vi "Dashboard Main.vi"() -> ()   [LabVIEW 2013]
uses:
  Vision Processing/TargetType.ctl
  <vilib>/event_ctls.llb/eventvkey.ctl
  <vilib>/Rock Robotics/WPI/Dashboard/WPI_DashboardLogging Global.vi
  <vilib>/Utility/config.llb/Write Key (String).vi
  <vilib>/Utility/config.llb/Write Key (I32).vi
  <vilib>/Utility/config.llb/NI_LVConfig.lvlib
panel:
  out "Image Message":string="Timeout in Camera Communications"
  in  "Rec Mode":enum32{"Stop", "Record", "Playback"}(radio)
  in  "Dashboard Tab":T1(tab)
  in  "Idle Loader":bool
  out "Charged":bool=TRUE
  out "60 PSI":bool
  out "PSI":dbl format="%#_3g"
  out "One Driver":bool
  out "120 PSI":bool
  out "Trigger Locked":bool=TRUE
  out "Reverse Drive":bool
  out "Robot Velocity (ft/s)":dbl(slide) scale=-20.0..20.0
  out "Gyro Mode":bool
  out "GREEN":bool
  out "YELLOW":bool
  out "RED":bool=TRUE
  out "Distance (ft)":dbl
  in  "Camera Settings":T2={"Frame Rate"=30, "Compression"=30, "Size"=1} {"Frame Rate" scale=1.0..30.0; "Size" items=["640x480", "320x240", "160x120"]}
  out "MotorSliders R":cluster{"MotorSlide1":dbl, "MotorSlide2":dbl} {"MotorSlide2" scale=-1.0..1.0 scale format="%#_2e"; "MotorSlide1" scale=-1.0..1.0 scale format="%#_2e"}
  out "MotorChart R":cluster{"Numeric":dbl, "Numeric":dbl}(graph)
  out "MotorSliders L":T3 {"MotorSlide4 2" scale=0.0..14.0 scale format="%#_2e"; "MotorSlide2" scale=-1.0..1.0 scale format="%#_2e"; "MotorSlide1" scale=-1.0..1.0 scale format="%#_2e"}
  out "MotorChart L":T4(graph)
  out "JS1 Z":dbl(slide) scale=-1.0..1.0 scale format="%#_2e"
  out "Joystick 1":cluster{"X":dbl, "Y":dbl}[](graph)
  out "JS Buttons 1":T5
  out "JS2 Z":dbl(slide) scale=-1.0..1.0 scale format="%#_2e"
  out "Joystick 2":cluster{"X":dbl, "Y":dbl}[](graph)
  out "JS Buttons 2":T5
  out "Mode":T6(ring)=enum."Auto Disabled"
  out "Camera IP":string
  in  "DB Camera Config":bool
  out "fps":dbl format="%#.1g"
  out "Mbps":dbl format="%#.1g"
  out "Mbps 2":bool
  out "Angular Rate":dbl
  out "Gyro Angle":dbl
  in  "Automatic or Timed":bool
  out "HOT OR NOT":bool
  in  "Score Limit":dbl=60.0
  in  "Color Components":T7={"Hue"={69.0, 101.0}, "Sat"={160.89285714285714, 255.0}, "Val"={36.42857142857143, 230.7142857142857}} {"Val" scale=0.0..255.0; "Sat" scale=0.0..255.0; "Hue" scale=0.0..255.0 scale format="%#_3g"}
  out "Distances":T9(array[cluster])
  in  "Test Slider":dbl(slide) scale=0.0..100.0 scale format="%#_3g"
  in  "On/Off":bool caption="Solenoid"
  in  "Test Name":u16(ring) items=["Select the test to run...", "Example Test", "-------------------------------", "List of tests is built in robot code.", "Replace with your own automated tests."]
  in  "Test Tree":string(tree)
  in  "Motor":cluster{"Value":dbl, "Enable":bool} {"Value" scale=-1.0..1.0 scale format="%#_3g"}
  out "Progress":T10 {"Test Progress" scale=0.0..100.0}
  in  "Rev/Fwd":cluster{"Forward":bool, "Reverse":bool}
  in  "Test Ring":u16(ring) items=["Auto", "Fixed indoor", "Fixed outdoor 1", "Fixed outdoor 2", "Fixed fluorescent 1", "Fixed fluorescent 2", "Hold current"]
  in  "Listbox":i32(listbox)
  out "Tree":string(tree)
  out "Camera Image":T11(plugin-control)
  in  "Enable Vision":bool=TRUE
  # "Left"
  # "Front"
  # "Right"
  # "Battery"
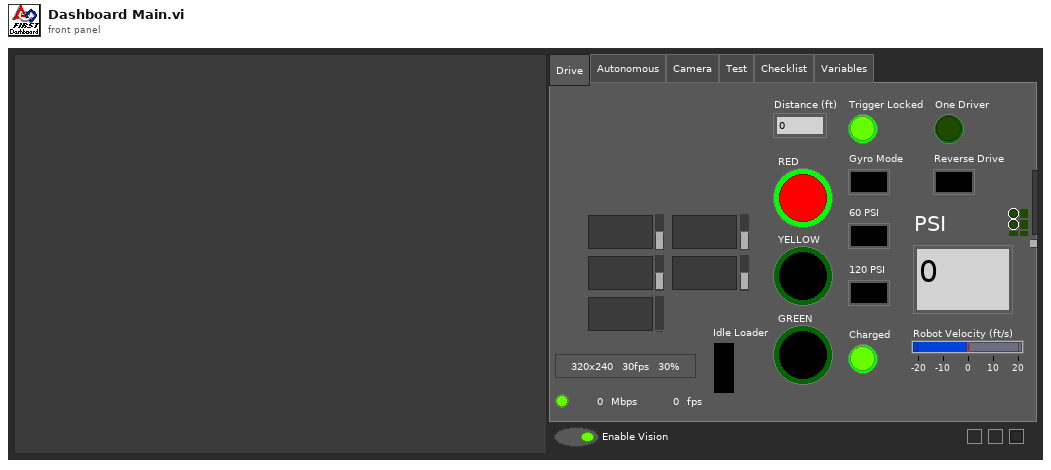
[diagram p1: front panel]
types:
  T1 = enum32{"Drive", "Autonomous", "Camera", "Test", "Checklist", "Variables"}
  T2 = cluster{"Frame Rate":i32, "Compression":i32, "Size":u16}
  T3 = cluster{"MotorSlide1":dbl, "MotorSlide2":dbl, "MotorSlide4 2":dbl}
  T4 = cluster{"Numeric":dbl, "Numeric":dbl, "Battery":sgl}
  T5 = cluster{bool, bool, bool, bool, bool, bool, bool, bool, bool, bool, bool, bool}
  T6 = enum8{"Tele-Op Disabled", "Tele-Op Enabled", "Auto Disabled", "Auto Enabled", "Test Disabled", "Test Enabled", ""}
  T7 = cluster{"Hue":cluster{dbl, dbl}, "Sat":cluster{dbl, dbl}, "Val":cluster{dbl, dbl}}
  T8 = typedef "TargetType.ctl" = enum16{"Not Hot", "Hot"}
  T9 = cluster{"Distance (ft)":dbl, "Target Center (-1 to 1)":cluster{"X":dbl, "Y":dbl}, "Left":bool, "State":T8}[]
  T10 = cluster{"Test Progress":u8, "Test Progress Text":string}
  T11 = typedef "IMAQ Image.ctl" = refnum<image>
  T12 = enum32{"Drive", "Operation", "Auto", "Test", "Checklist", "Variables"}
  T13 = typedef "Image Type" = u32
  T14 = cluster{"Digital Inputs":bool[], "Digital Outputs":bool[]}
  T15 = cluster{"Competition mode":bool, "Robot Link":bool, "Autonomous":bool, "Enabled":bool, "E-Stop":bool, "Simulated":bool, "TestMode":bool, "Docked Window":bool}
  T16 = cluster{"Boolean Array[0]":bool, "Boolean Array[1]":bool, "Boolean Array[2]":bool, "Boolean Array[3]":bool, "Boolean Array[4]":bool, "Boolean Array[5]":bool, "Boolean Array[6]":bool, "Boolean Array[7]":bool, "Boolean Array[8]":bool, "Boolean Array[9]":bool, "Boolean Array[10]":bool, "Boolean Array[11]":bool}
  T17 = cluster{cluster{dbl, dbl}, cluster{dbl, dbl}, cluster{dbl, dbl}}
  T18 = cluster{"Horizontal":bool, "Aspect Score":dbl, "Rect Score":dbl, cluster{"Left":dbl, "Top":dbl, "Right":dbl, "Bottom":dbl}, "Equiv H":dbl, "Equiv V":dbl}[]
  T19 = cluster{"Scores":cluster{"Total":dbl, "Left":dbl, "Right":dbl, "Ratio":dbl, "Vertical":dbl, "index":i32, "State":T8}, "Verticals":cluster{"Horizontal?":bool, "Aspect Score":dbl, "Rect Score":dbl, cluster{"Left":dbl, "Top":dbl, "Right":dbl, "Bottom":dbl}, "Equiv H":dbl, "Equiv V":dbl}, "Horizontals":cluster{"Horizontal?":bool, "Aspect Score":dbl, "Rect Score":dbl, cluster{"Left":dbl, "Top":dbl, "Right":dbl, "Bottom":dbl}, "Equiv H":dbl, "Equiv V":dbl}, "Validated":bool}[]
  T20 = cluster{"Scores":cluster{"Total":dbl, "Left":dbl, "Right":dbl, "Ratio":dbl, "Vertical":dbl, "index":i32, "State":T8}, "Verticals":cluster{"Horizontal?":bool, "Aspect Score":dbl, "Rect Score":dbl, cluster{"Left":dbl, "Top":dbl, "Right":dbl, "Bottom":dbl}, "Equiv H":dbl, "Equiv V":dbl}, "Horizontals":cluster{"Horizontal?":bool, "Aspect Score":dbl, "Rect Score":dbl, cluster{"Left":dbl, "Top":dbl, "Right":dbl, "Bottom":dbl}, "Equiv H":dbl, "Equiv V":dbl}, "Distance (ft)":dbl, "Target Center (-1 to 1)":cluster{"X":dbl, "Y":dbl}}[]
  T21 = cluster{"Distance (ft)":dbl, "Target Center (-1 to 1)":cluster{"X":dbl, "Y":dbl}, "Left":bool, "State":T8}
  T22 = typedef "NI_LVConfig.lvlib/Config Data RefNum.ctl" = refnum<k1>
  T23 = typedef "eventvkey.ctl" = enum16{"ASCII", "Enter", "Return", "Shift", "Ctrl", "Alt", "Cmd", "Opt", "Caps", "NumLock", "Clear", "Break", "Up", "Down", "Left", "Right", "Insert", "Delete", "Home", "End", "PageUp", "PageDown", "Escape", "Help", "Pause", "ScrollLock", "F1", "F2", "F3", "F4", "F5", "F6", "F7", "F8", "F9", "F10", "F11", "F12", "F13", "F14", "F15", "F16", "F17", "F18", "F19", "F20", "F21", "F22", "F23", "F24", "Play", "VolumeUp", "VolumeDown", "Mute", "Two Byte Char"}
  T24 = cluster{"Image Size":bool, "Image Type":bool, "Pixel Value":bool, "ROI Information":bool, "Zoom Factor":bool}
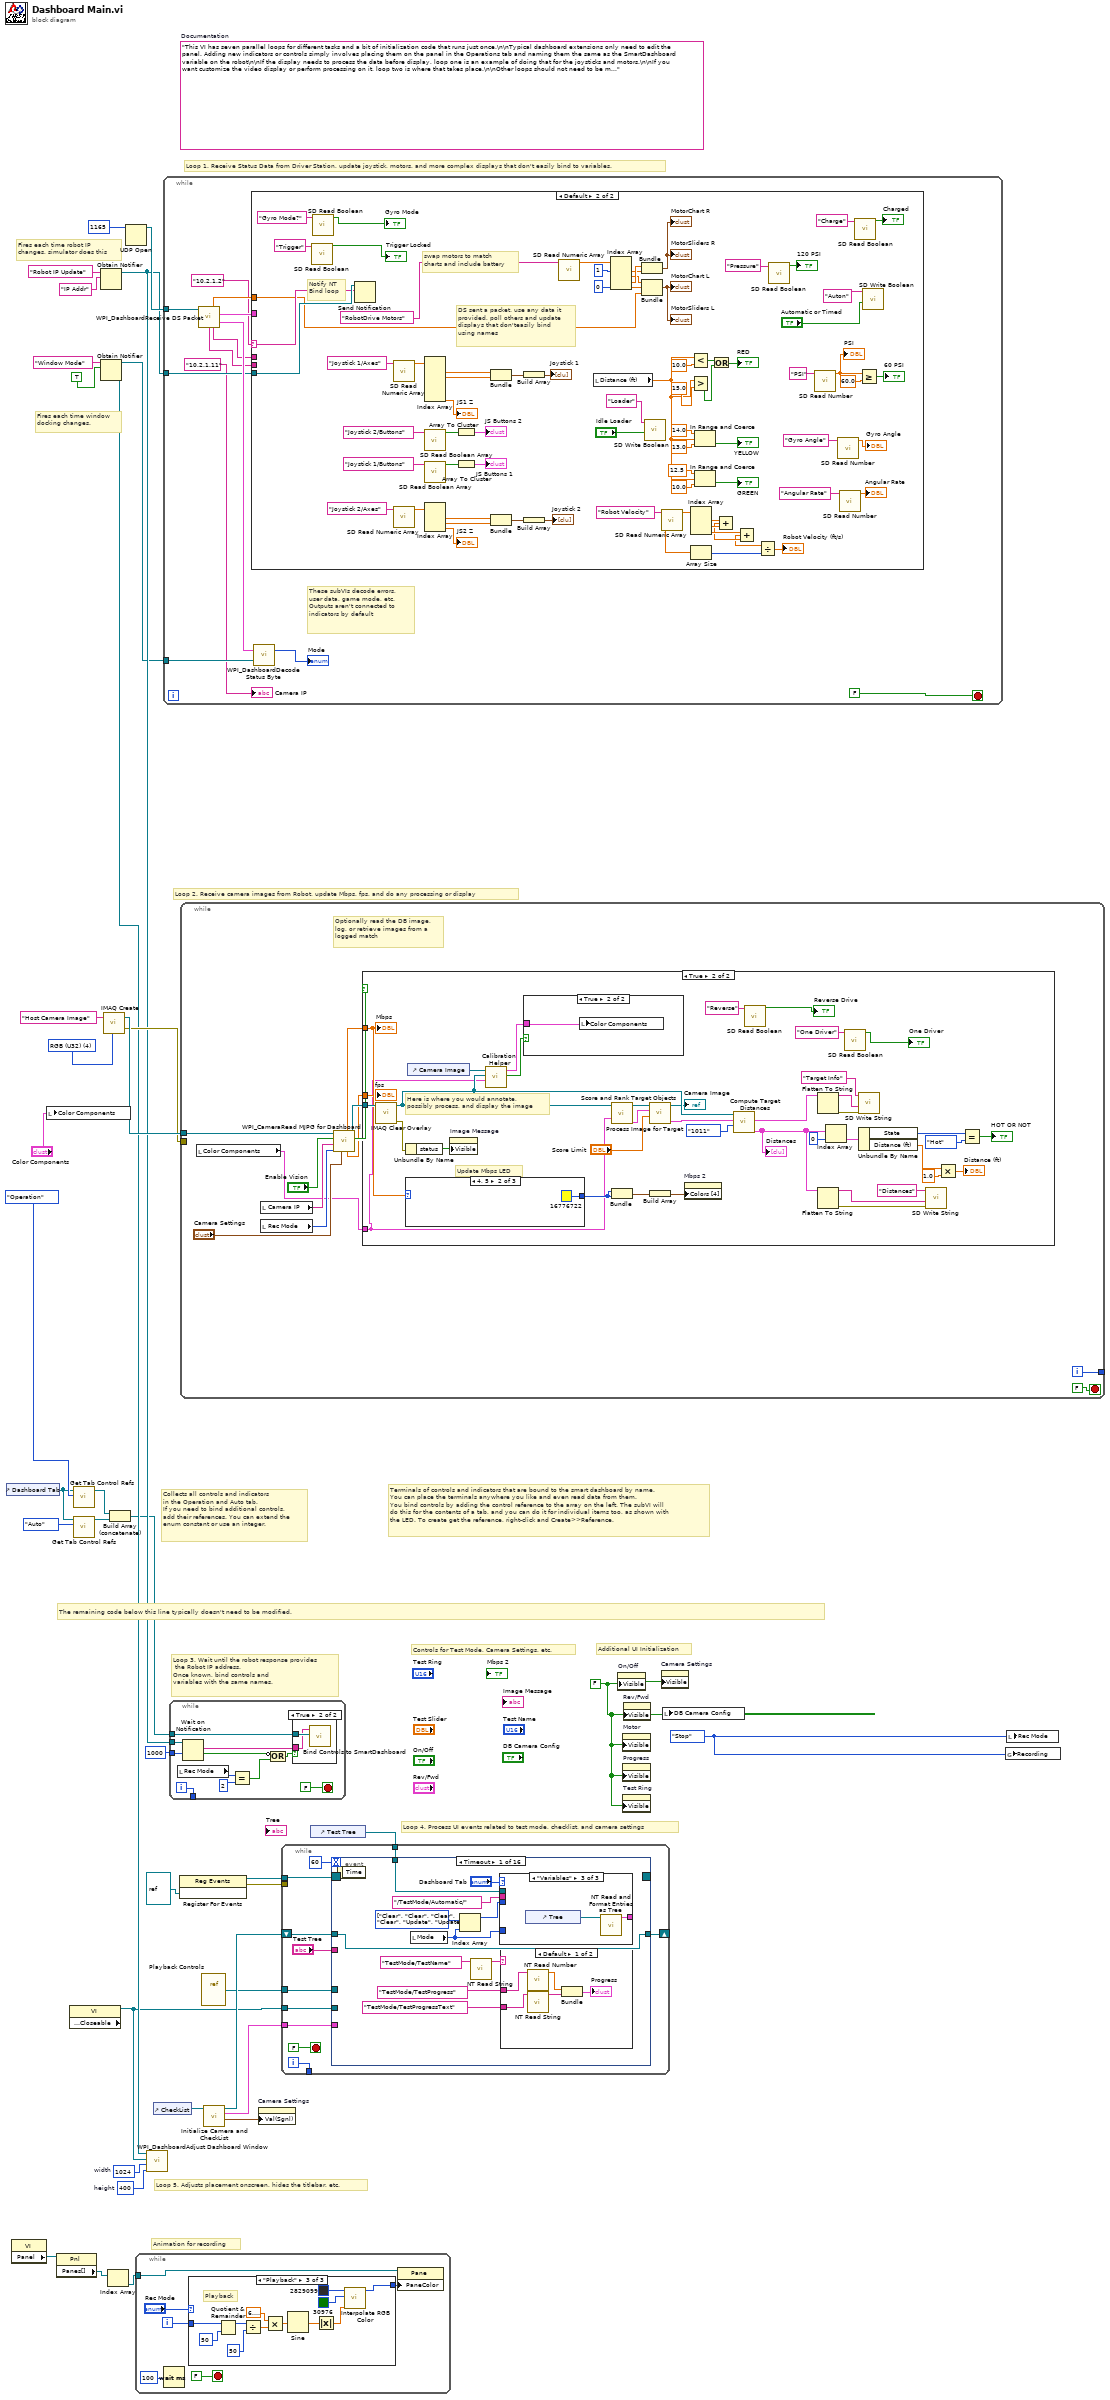
[diagram p0: block diagram]
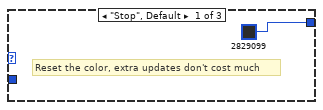
[diagram p2: hidden frame]
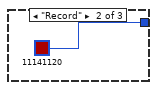
[diagram p3: hidden frame]
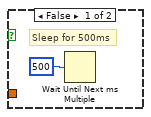
[diagram p5: hidden frame]
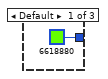
[diagram p7: hidden frame]
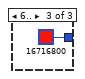
[diagram p8: hidden frame]
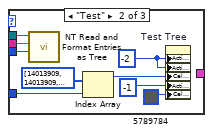
[diagram p10: hidden frame]
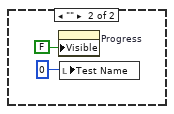
[diagram p11: hidden frame]
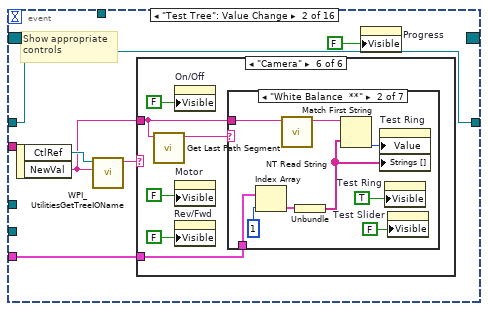
[diagram p12: hidden frame]
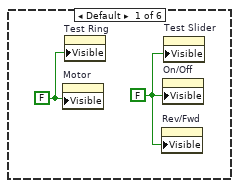
[diagram p13: hidden frame]
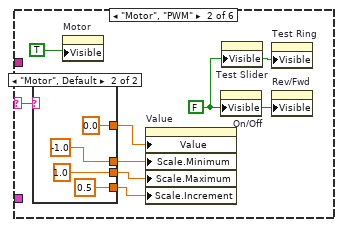
[diagram p14: hidden frame]
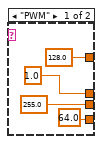
[diagram p15: hidden frame]
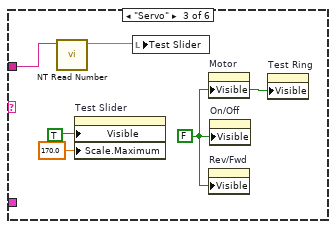
[diagram p16: hidden frame]
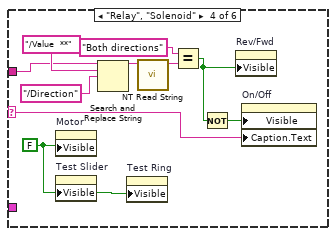
[diagram p17: hidden frame]
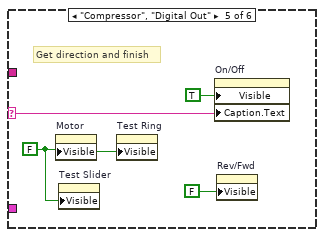
[diagram p18: hidden frame]
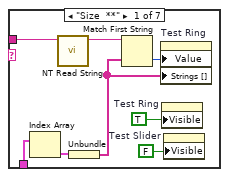
[diagram p19: hidden frame]
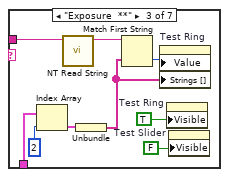
[diagram p20: hidden frame]
diagram:
  w8 = enum32{"Stop", "Record", "Playback"}."Stop" ("Rec Mode")
  w11 = 400  # height
  w12 = 1024  # width
  w25 = FALSE ("Visible")
  (unwired) "This VI has seven parallel loops for different tasks and a bit of initialization code that runs just once.\n\nTypical dashboard extensions only need to edit the panel. Adding new indicators or controls simply involves placing them on the panel in the Operations tab and naming them the same as the SmartDashboard variable on the robot\n\nIf the display needs to process the data before display, loop one is an example of doing that for the joysticks and motors.\n\nIf you want customize the video display or perform processing on it, loop two is where that takes place.\n\nOther loops should not need to be modified. They are pretty standard, and document the task they perform."  # Documentation
  w35 = T13 4 items=["Grayscale (U8)", "Grayscale (I16)", "Grayscale (SGL)", "Complex (CSG)", "RGB (U32)", "HSL (U32)", "RGB (U64)"] ("Image Type")
  # "Controls for Test Mode, Camera Settings, etc."
  # "Additional UI Initialization"
  # "Animation for recording"
  # "Fires each time robot IP\nchanges, simulator does this"
  # "Fires each time window\ndocking changes."
  # "Collects all controls and indicators\nin the Operation and Auto tab.\nIf you need to bind additional controls,\nadd their references. You can extend the\nenum constant or use an integer."
  # "The remaining code below this line typically doesn't need to be modified."
  # "Loop 4. Process UI events related to test mode, checklist, and camera settings"
  # "Terminals of controls and indicators that are bound to the smart dashboard by name.\nYou can place the terminals anywhere you like and even read data from them.\nYou bind controls by adding the control reference to the array on the left. The subVI will\ndo this for the contents of a tab, and you can do it for individual items too, as shown with\nthe LED. To create get the reference, right-click and Create>>Reference."
  # "Loop 3. Wait until the robot response provides\n the Robot IP address.\nOnce known, bind controls and\nvariables with the same names."
  # "Loop 5. Adjusts placement onscreen, hides the titlebar, etc."
  # "Loop 1. Receive Status Data from Driver Station, update joystick, motors, and more complex displays that don't easily bind to variables."
  # "Loop 2. Receive camera images from Robot, update Mbps, fps, and do any processing or display"
  n1 = control-ref of="Dashboard Tab"() -> (w6:refnum<vi>)
  n2 = property class="VI"() -> ("Panel"=w19:refnum<vi>)  [unwired: 2 in, 2 out]
  n3 = local write "Color Components"("Color Components") -> ()
  n4 = property class="Pnl"(reference=w19) -> ("Panes[]"=w20:refnum<vi>[])  [unwired: 1 in, 2 out]
  n5 = property class="VI" props=["Front Panel.Closeable"]() -> (reference out=w7:refnum<vi>)  [unwired: 2 in, 2 out]
  n6 = call <vilib>:"Get Tab Control Refs.vi"("Page Index"=T12."Operation" ("Dashboard Tab"), "TabControl in"=w6) -> ("ControlsOnPage"=w4:refnum<vi>[])  [unwired: 9 in]
  n7 = call <vilib>:"Get Tab Control Refs.vi"("Page Index"=T12."Auto" ("Dashboard Tab"), "TabControl in"=w6) -> ("ControlsOnPage"=w5:refnum<vi>[])  [unwired: 9 in]
  n8 = Obtain Notifier(name (unnamed)="Robot IP Update", notification data type="IP Addr" ("name (unnamed)")) -> (notifier out=w29:refnum<notifier>)  [unwired: 2 in, 2 out]
  n9 = Obtain Notifier(name (unnamed)="Window Mode", notification data type=TRUE) -> (notifier out=w10:refnum<notifier>)  [unwired: 2 in, 2 out]
  n10 = call "IMAQ Create"("Image Name"="Host Camera Image", "Image Type"=w35) -> ("New Image"=w33:T11, "error out"=w32:errorcluster)  [unwired: 2 in, 1 out]
  n11 = Index Array(array=w20) -> (element=w18:refnum<vi>)  [unwired: 1 in]
  n12 = Build Array (concatenate)(w4, w5) -> (w3:refnum<vi>[])
  n13 = UDP Open(11:u16 1165 ("port")) -> (port=w36:refnum<k16>)  [unwired: 2 in, 4 out]
  n14 = while {
    tunnel: w18 -> [w39]
    i -> [w42]
    stop <- FALSE stop-if-true
    n15 = Wait (ms)(milliseconds to wait=u32 100) -> ()  [unwired: 1 out]
    n16 = case shown="\"Playback\"" "Rec Mode" {
      tunnel: w42 -> [_ _ w57]
      tunnel: [u32 2829099 ("Base Color") u32 11141120 ("Target Color") w46] -> w38
      frame "Stop", Default {
        # "Reset the color, extra updates don't cost much"
      }
      frame "Record" {
      }
      frame "Playback" {
        # "Playback"
        n17 = Quotient & Remainder(x=w57, y=u32 50 ("milliseconds to wait")) -> (x-y*floor(x/y)=w53:u32)  [unwired: 1 out]
        n18 = Divide(x=w53, y=u32 50 ("milliseconds to wait")) -> (x/y=w50:dbl)
        n19 = Multiply(x=6.283185307179586, y=w50) -> (x*y=w55:dbl)
        n20 = Sine(x=w55) -> (sin(x)=w54:dbl)
        n21 = Absolute Value(x=w54) -> (abs(x)=w47:dbl)
        n22 = call "Interpolate RGB Color.vi"("Proportion"=w47, "Target Color"=u32 30976, "Base Color"=u32 2829099) -> ("Result Color"=w46:u32)  [unwired: 8 in]
      }
    }
    n23 = property class="Pane"(reference=w39, "PaneColor"=w38) -> ()  [unwired: 1 in, 2 out]
  }
  n24 = call <vilib>:"WPI_DashboardAdjust Dashboard Window.vi"("height"=w11, "width"=w12, "reference in"=w7, "Notifier in"=w10) -> ()  [unwired: 8 in]
  n25 = control-ref of="CheckList"() -> (w9:refnum<vi>)
  n26 = while {
    tunnel: w36 -> [w67]
    tunnel: w29 -> [w64]
    tunnel: w10 -> [w66]
    stop <- FALSE stop-if-true
    # "These subVIs decode errors, user data, game mode, etc.\nOutputs aren't connected to indicators by default"
    n27 = call <vilib>:"WPI_DashboardReceive DS Packet.vi"("Recv Socket"=w67) -> ("Battery"=w60:sgl, "Driver Station"=w61:T14, "Status"=w68:T15, "Low Priority User Data"=w63:string, "High Priority User Data"=w62:string)  [unwired: 1 in, 9 out]
    n28 = case shown="Default" "10.2.1.2" {
      selector: "10.2.1.2" -> [_ w121]
      tunnel: w64 -> [_ w122]
      tunnel: w63 -> [_ _]
      tunnel: w62 -> [_ _]
      tunnel: w61 -> [_ _]
      tunnel: w60 -> [_ w120]
      frame "0.0.0.0" {
        # "DS not sending packets, or no robot exists yet.\nDon't poll the variables"
      }
      frame Default {
        # "Notify NT\nBind loop"
        # "DS sent a packet. use any data it\nprovided, poll others and update\ndisplays that don'teasily bind\nusing names"
        # "swap motors to match\ncharts and include battery"
        n29 = call <vilib>:"SD Read Boolean.vi"("Name"="Trigger") -> ("Boolean"=→"Trigger Locked":bool)  [unwired: 8 in, 2 out]
        n30 = call <vilib>:"SD Read Boolean.vi"("Name"="Gyro Mode?") -> ("Boolean"=→"Gyro Mode":bool)  [unwired: 8 in, 2 out]
        n31 = Send Notification(notification=w121, notifier=w122) -> ()  [unwired: 1 in, 2 out]
        n32 = call <vilib>:"SD Read Numeric Array.vi"("Name"="Joystick 1/Axes") -> ("Numeric Array"=w138:dbl[])  [unwired: 8 in, 2 out]
        n33 = call <vilib>:"SD Read Numeric Array.vi"("Name"="Joystick 2/Axes") -> ("Numeric Array"=w132:dbl[])  [unwired: 8 in, 2 out]
        n34 = Index Array(array=w138) -> (element #1=w135:dbl, element #2=w136:dbl, element #3=→"JS1 Z":dbl)  [unwired: 6 in, 3 out]
        n35 = call <vilib>:"SD Read Boolean Array.vi"("Name"="Joystick 2/Buttons") -> ("Boolean Array"=w131:bool[])  [unwired: 8 in, 2 out]
        n36 = call <vilib>:"SD Read Boolean Array.vi"("Name"="Joystick 1/Buttons") -> ("Boolean Array"=w140:bool[])  [unwired: 8 in, 2 out]
        n37 = Index Array(array=w132) -> (element #1=w127:dbl, element #2=w126:dbl, element #3=→"JS2 Z":dbl)  [unwired: 3 in]
        n38 = Array To Cluster(array=w131) -> (cluster=→"JS Buttons 2":T16)
        n39 = Array To Cluster(array=w140) -> (cluster=→"JS Buttons 1":T16)
        n40 = Bundle("Numeric"=w135, "Numeric"=w136) -> (w134:cluster{"Numeric":dbl, "Numeric":dbl})  [unwired: 1 in]
        n41 = Bundle("Numeric"=w127, "Numeric"=w126) -> (w128:cluster{"Numeric":dbl, "Numeric":dbl})  [unwired: 1 in]
        n42 = Build Array(w134) -> (→"Joystick 1":cluster{"Numeric":dbl, "Numeric":dbl}[])
        n43 = Build Array(w128) -> (→"Joystick 2":cluster{"Numeric":dbl, "Numeric":dbl}[])
        n44 = call <vilib>:"SD Read Numeric Array.vi"("Name"="RobotDrive Motors") -> ("Numeric Array"=w119:dbl[])  [unwired: 8 in, 2 out]
        n45 = local read "Distance (ft)"() -> (w100:dbl)
        n46 = Index Array(array=w119, index #1=1, index #4=0) -> (element #1=w115:dbl, element #2=w114:dbl, element #3=w116:dbl, element #4=w111:dbl)  [unwired: 2 in]
        n47 = Bundle("Numeric"=w116, "Numeric"=w115) -> (→"MotorChart R" →"MotorSliders R":cluster{"Numeric":dbl, "Numeric":dbl})  [unwired: 1 in]
        n48 = Bundle("Numeric"=w114, "Numeric"=w111, "Battery"=w120) -> (→"MotorChart L" →"MotorSliders L":T4)  [unwired: 1 in]
        n49 = call <vilib>:"SD Write Boolean.vi"("Boolean"="Idle Loader", "Name"="Loader") -> ()  [unwired: 8 in, 2 out]
        n50 = call <vilib>:"SD Read Numeric Array.vi"("Name"="Robot Velocity") -> ("Numeric Array"=w95:dbl[])  [unwired: 8 in, 2 out]
        n51 = Less?(x=w100, y=10.0 ("x")) -> (x < y?=w99:bool)
        n52 = Greater?(x=w100, y=15.0 ("x")) -> (0:w98:bool)
        n53 = Index Array(array=w95) -> (element #1=w94:dbl, element #2=w93:dbl, element #3=w92:dbl)  [unwired: 3 in]
        n54 = Array Size(array=w95) -> (size(s)=w89:i32)
        n55 = In Range and Coerce(upper limit=14.0, x=w100, lower limit=13.0) -> (In Range?=→"YELLOW":bool)  [unwired: 1 out]
        n56 = In Range and Coerce(upper limit=12.5, x=w100, lower limit=10.0) -> (In Range?=→"GREEN":bool)  [unwired: 1 out]
        n57 = Or(x=w99, y=w98) -> (x .or. y?=→"RED":bool)
        n58 = Add(x=w94, y=w93) -> (x+y=w91:dbl)
        n59 = Add(x=w92, y=w91) -> (x+y=w90:dbl)
        n60 = Divide(x=w90, y=w89) -> (x/y=→"Robot Velocity (ft/s)":dbl)
        n61 = call <vilib>:"SD Read Boolean.vi"("Name"="Pressure") -> ("Boolean"=→"120 PSI":bool)  [unwired: 8 in, 2 out]
        n62 = call <vilib>:"SD Read Number.vi"("Name"="PSI") -> ("Numeric"=w81:dbl)  [unwired: 8 in, 2 out]
        "PSI" <- w81
        n63 = call <vilib>:"SD Read Number.vi"("Name"="Gyro Angle") -> ("Numeric"=→"Gyro Angle":dbl)  [unwired: 8 in, 2 out]
        n64 = call <vilib>:"SD Read Number.vi"("Name"="Angular Rate") -> ("Numeric"=→"Angular Rate":dbl)  [unwired: 8 in, 2 out]
        n65 = call <vilib>:"SD Read Boolean.vi"("Name"="Charge") -> ("Boolean"=→"Charged":bool)  [unwired: 8 in, 2 out]
        n66 = Greater Or Equal?(x=w81, y=60.0) -> (x >= y?=→"60 PSI":bool)
        n67 = call <vilib>:"SD Write Boolean.vi"("Boolean"="Automatic or Timed", "Name"="Auton") -> ()  [unwired: 8 in, 2 out]
      }
    }
    n68 = call <vilib>:"WPI_DashboardDecode Status Byte.vi"("Window Mode Notifier"=w66, "Status"=w68) -> ("Mode"=→"Mode":T6)  [unwired: 1 out]
    "Camera IP" <- "10.2.1.11" ("Camera IP")
  }
  n69 = while {
    tunnel: w3 -> [w154]
    tunnel: w29 -> [w152]
    tunnel: [w150] -> _
    tunnel: u32 1000 ("milliseconds to wait") -> [w149]
    i -> [w150]
    stop <- FALSE stop-if-true
    n70 = local read "Rec Mode"() -> (w145:enum32{"Stop", "Record", "Playback"})
    n71 = Wait on Notification(notifier=w152, timeout in ms (-1)=w149) -> (notification=w151:string, timed out?=w147:bool)  [unwired: 2 in, 2 out]
    n72 = Equal?(x=w145, y=u16 2 ("Rec Mode")) -> (x = y?=w146:bool)
    n73 = Compound Arithmetic op=OR(invert w147, w146) -> (w148:bool)
    n74 = case shown="True" w148 {
      tunnel: w154 -> [_ w156]
      tunnel: w151 -> [_ w155]
      frame False {
      }
      frame True {
        n75 = call <vilib>:"Bind Controls to SmartDashboard.vi"("Bound Control Refs"=w156, "Server IP Address"=w155) -> ()  [unwired: 10 in]
      }
    }
  }
  n76 = register-events(refnum<vi> refnum) -> (reference out=w16:refnum<event-registration>, error out=w15:errorcluster)  [unwired: 2 in]
  n77 = while {
    tunnel: w33 -> [w166]
    tunnel: w32 -> [_]
    tunnel: [w167] -> _
    i -> [w167]
    stop <- FALSE stop-if-true
    # "Optionally read the DB image,\nlog, or retrieve images from a\nlogged match"
    n78 = local read "Color Components"() -> (w157:T7)
    n79 = local read "Camera IP"() -> (w159:string)
    n80 = local read "Rec Mode"() -> (w158:enum32{"Stop", "Record", "Playback"})
    n81 = call <vilib>:"WPI_CameraRead MJPG for Dashboard.vi"("Camera Settings"="Camera Settings", "Rec Mode"=w158, "Camera IP"=w159, "Enable"="Enable Vision", "Refnum in"=w166) -> ("Active"=w163:bool, "Refnum out"=w165:T11, "FPS"=w162:dbl, "Bandwidth (Mbps)"=w161:dbl)  [unwired: 3 in]
    n82 = case shown="True" w163 {
      tunnel: w165 -> [_ w203]
      tunnel: w161 -> [_ w202]
      tunnel: w162 -> [_ w201]
      tunnel: w157 -> [_ w179]
      frame False {
        # "Sleep for 500ms"
        n83 = Wait Until Next ms Multiple(millisecond multiple=u32 500) -> ()  [unwired: 1 out]
      }
      frame True {
        # "Here is where you would annotate,\npossibly process, and display the image"
        # "Update Mbps LED"
        n84 = call "IMAQ Clear Overlay"("Image"=w203) -> ("error out"=w207:errorcluster, "Image Out"=w183:T11)  [unwired: 2 in, 7 out]
        n85 = Unbundle By Name(w207) -> ("status"=w208:bool)
        n86 = case shown="4, 5" w202 {
          tunnel: [u32 6618880 ("Color Box") u32 16776722 ("Color Box") u32 16716800 ("Color Box")] -> w204
          frame Default {
          }
          frame 4, 5 {
          }
          frame 6.. {
          }
        }
        n87 = control-ref of="Camera Image"() -> (w195:refnum<vi>)
        n88 = property on="Image Message" class="Str"("Visible"=w208) -> ()  [unwired: 2 in, 2 out]
        n89 = call "Calibration Helper.vi"("Color Components"=w179, "Image"=w183, "Image Ctl Refnum"=w195) -> ("Changed"=w180:bool, "output color"=w181:T17)  [unwired: 7 in]
        n90 = case shown="True" w180 {
          tunnel: w181 -> [_ w209]
          frame False {
          }
          frame True {
            n91 = local write "Color Components"(w209) -> ()
          }
        }
        n92 = call "Process Image for Target.vi"("Src Image"=w183, "Color Components"=w179) -> ("Src Image Out"=w200:T11, "Particles"=w199:T18)  [unwired: 11 in, 1 out]
        n93 = Bundle("Color Box"=w204, "Color Box"=w204) -> (w206:cluster{"Color Box":u32, "Color Box":u32})  [unwired: 1 out]
        n94 = call "Score and Rank Target Objects.vi"("Score Limit"="Score Limit", "Particles"=w199, "Image in"=w200) -> ("Target Info"=w198:T19, "Annotated Image"=→"Camera Image":T11)  [unwired: 7 in]
        n95 = Build Array(w206) -> (w205:cluster{"Color Box":u32, "Color Box":u32}[])
        n96 = property on="Mbps 2" class="Bool (strict)"("Colors [4]"=w205) -> ()  [unwired: 2 in, 2 out]
        n97 = call "Compute Target Distances.vi"("Camera Type"=enum16{"206", "1011", "1013"}."1011", "Target Info"=w198, "Image in"=w183) -> ("Distances"=w174:T9, "Target Info"=w175:T20)  [unwired: 6 in, 1 out]
        "Distances" <- w174
        n98 = call <vilib>:"SD Read Boolean.vi"("Name"="Reverse") -> ("Boolean"=→"Reverse Drive":bool)  [unwired: 8 in, 2 out]
        n99 = Flatten To String(anything=w175) -> (data string=w190:string, error out=w191:errorcluster)  [unwired: 3 in, 1 out]
        n100 = Flatten To String(anything=w174) -> (data string=w192:string, error out=w194:errorcluster)  [unwired: 3 in, 1 out]
        n101 = Index Array(array=w174, index=0) -> (element=w187:T21)
        n102 = call <vilib>:"SD Read Boolean.vi"("Name"="One Driver") -> ("Boolean"=→"One Driver":bool)  [unwired: 8 in, 2 out]
        n103 = call <vilib>:"SD Write String.vi"("error in"=w191, "String"=w190, "Name"="Target Info") -> ()  [unwired: 7 in, 2 out]
        n104 = Unbundle By Name(w187) -> ("State"=w178:T8, "Distance (ft)"=w185:dbl)
        n105 = call <vilib>:"SD Write String.vi"("error in"=w194, "String"=w192, "Name"="Distances") -> ()  [unwired: 7 in, 2 out]
        n106 = Multiply(x=w185, y=1.0) -> (x*y=→"Distance (ft)":dbl)
        n107 = Equal?(x=w178, y=TargetType."Hot") -> (x = y?=→"HOT OR NOT":bool)
        "Mbps" <- w202
        "fps" <- w201
      }
    }
  }
  n108 = vi-ref "Playback Controls.vi"() -> (w17:refnum<vi>)
  n109 = call "Initialize Camera and CheckList.vi"("ListBox in"=w9) -> ("Cluster"=w23:cluster{"value":i32, "value":i32, "index":i32}, "Array"=w24:cluster{string[]}[], "File Refnum"=w22:T22)  [unwired: 8 in]
  n110 = property on="Camera Settings" class="Clust (strict)"("Val(Sgnl)"=w23) -> ()  [unwired: 2 in, 2 out]
  n111 = control-ref of="Test Tree"() -> (w21:refnum<vi>)
  n112 = while {
    tunnel: w24 -> [w220]
    shift-right: [w219] -> _
    shift-left: w22 -> [w218]
    tunnel: [w217] -> _
    tunnel: w21 -> [w216]
    tunnel: w17 -> [w215]
    tunnel: w16 -> [w214]
    tunnel: w15 -> [_]
    tunnel: w7 -> [w213]
    i -> [w217]
    stop <- FALSE stop-if-true
    n113 = event shown="[0] Timeout" {
      selector: w214 -> [_ _ _ _ _ _ _ _ _ _ _ _ _ _ _ _]
      dyn-events: [_ _ _ _ _ _ _ _ _ _ _ _ _ w458 _ _] -> _
      timeout: u32 60 ("milliseconds to wait") -> [_ _ _ _ _ _ _ _ _ _ _ _ _ _ _ _]
      tunnel: w216 -> [w230 _ _ _ _ _ _ _ _ _ _ _ _ _ _ _]
      tunnel: "Test Tree" -> [_ _ _ _ _ _ _ _ w427 w435 w437 w441 w449 _ _ _]
      tunnel: w220 -> [_ w254 _ _ _ _ w391 w421 _ _ _ _ _ _ _ _]
      tunnel: [w224 w253 w352 w357 w365 w377 w390 w414 w426 w433 w436 w440 w448 w460 w474 w475] -> w219
      tunnel: w218 -> [w224 w253 w352 w357 w365 w377 w389 w414 w426 w433 w436 w440 w448 w460 w474 w475]
      tunnel: w215 -> [_ _ _ _ _ _ _ _ _ _ _ _ _ w461 _ w478]
      tunnel: w213 -> [_ _ _ _ _ _ _ _ _ _ _ _ _ w456 _ _]
      event Timeout {
        w229 = enum16{"Update", "Clear"}[] [enum."Clear", enum."Clear", enum."Clear", enum."Clear", enum."Update", enum."Update", enum."Clear"] items=["Update", "Clear"]
        n114 = event-data() -> ()  [unwired: 1 in, 1 out]
        n115 = local read "Mode"() -> (w227:T6)
        n116 = Index Array(array=w229, index=w227) -> (element=w228:enum16{"Update", "Clear"})
        n117 = call <vilib>:"NT Read String.vi"("Name"="TestMode/TestName") -> ("String"=w233:string)  [unwired: 9 in, 1 out]
        n118 = case shown="\"Variables\"" "Dashboard Tab" {
          tunnel: w230 -> [_ w243 _]
          tunnel: "/TestMode/Automatic/" ("Name Pattern") -> [_ w242 _]
          tunnel: w228 -> [_ w241 _]
          tunnel: w227 -> [_ w239 _]
          tunnel: [_ _ w245] -> _
          frame "Autonomous", Default {
          }
          frame "Test" {
            w238 = -2 ("Active Item:Row Number")
            n119 = call <vilib>:"NT Read and Format Entries as Tree.vi"("Operation"=w241, "Name Pattern"=w242, "Tree Refnum"=w243) -> ()  [unwired: 7 in, 2 out]
            n120 = Index Array(array=u32[] [14013909, 14013909, 14013909, 14013909, 14013909, 16777215, 14013909], index=w239) -> (element=w237:u32)
            n121 = property on="Test Tree" class="Tree (strict)"("Active Item Row Number"=w238, "ActiveColNum"=w238, "CellBG"=w237, "Active Item Row Number"=-1 ("Active Item:Row Number"), "CellBG"=u32 5789784 ("Color Box")) -> ()  [unwired: 2 in, 2 out]
          }
          frame "Variables" {
            n122 = control-ref of="Tree"() -> (w244:refnum<vi>)
            n123 = call <vilib>:"NT Read and Format Entries as Tree.vi"("Tree Refnum"=w244) -> ("Formatted Strings"=w245:cluster{"Name":string, "Value":string}[])  [unwired: 9 in, 1 out]
          }
        }
        n124 = case shown="Default" w233 {
          tunnel: "TestMode/TestProgress" ("Name") -> [w247 _]
          tunnel: "TestMode/TestProgressText" ("Name") -> [w246 _]
          frame Default {
            n125 = call <vilib>:"NT Read Number.vi"("Name"=w247) -> ("Numeric"=w248:dbl)  [unwired: 9 in, 1 out]
            n126 = call <vilib>:"NT Read String.vi"("Name"=w246) -> ("String"=w249:string)  [unwired: 9 in, 1 out]
            n127 = Bundle("Numeric"=w248, "String"=w249) -> (→"Progress":cluster{"Numeric":dbl, "String":string})  [unwired: 1 in]
          }
          frame "" {
            n128 = property on="Progress" class="Clust (strict)"("Visible"=FALSE) -> ()  [unwired: 2 in, 2 out]
            n129 = local write "Test Name"(u16 0) -> ()
          }
        }
      }
      event "Test Tree": Value Change {
        # "Show appropriate\ncontrols"
        n130 = event-data() -> ("CtlRef"=w257:refnum<vi>, "NewVal"=w255:string)  [unwired: 1 in]
        n131 = call <vilib>:"WPI_UtilitiesGetTreeIOName.vi"("NewVal"=w255, "TreeControl in"=w257) -> ("I/O Name"=w258:string)  [unwired: 9 in]
        n132 = case shown="\"Camera\"" w258 {
          selector: w258 -> [_ w265 _ w283 w292 _]
          tunnel: w255 -> [_ _ w280 w282 _ w299]
          tunnel: w254 -> [_ _ _ _ _ w298]
          frame Default {
            w260 = FALSE ("Visible")
            w259 = FALSE ("Visible")
            n133 = property on="Motor" class="Clust (strict)"("Visible"=w259) -> ()  [unwired: 2 in, 2 out]
            n134 = property on="Test Ring" class="Ring (strict)"("Visible"=w259) -> ()  [unwired: 2 in, 2 out]
            n135 = property on="Rev/Fwd" class="Clust (strict)"("Visible"=w260) -> ()  [unwired: 2 in, 2 out]
            n136 = property on="On/Off" class="Bool (strict)"("Visible"=w260) -> ()  [unwired: 2 in, 2 out]
            n137 = property on="Test Slider" class="Slide (strict)"("Visible"=w260) -> ()  [unwired: 2 in, 2 out]
          }
          frame "Motor", "PWM" {
            w266 = FALSE ("Visible")
            n138 = case shown="\"Motor\", Default" w265 {
              tunnel: [1.0 ("Value") -1.0 ("Value")] -> w264
              tunnel: [255.0 ("Value") 1.0 ("Value")] -> w263
              tunnel: [128.0 ("Value") 0.0 ("Value")] -> w262
              tunnel: [64.0 ("Value") 0.5 ("Value")] -> w261
              frame "PWM" {
              }
              frame "Motor", Default {
              }
            }
            n139 = property on="Motor" class="Clust (strict)"("Visible"=TRUE) -> ()  [unwired: 2 in, 2 out]
            n140 = property on="Value" class="Slide (strict)"("Value"=w262, "Scale.Minimum"=w264, "Scale.Maximum"=w263, "Scale.Increment"=w261) -> ()  [unwired: 2 in, 2 out]
            n141 = property on="On/Off" class="Bool (strict)"("Visible"=w266) -> ()  [unwired: 2 in, 2 out]
            n142 = property on="Test Slider" class="Slide (strict)"("Visible"=w266) -> ()  [unwired: 2 in, 2 out]
            n143 = property on="Test Ring" class="Ring (strict)"("Visible"=w266) -> ()  [unwired: 2 in, 2 out]
            n144 = property on="Rev/Fwd" class="Clust (strict)"("Visible"=w266) -> ()  [unwired: 2 in, 2 out]
          }
          frame "Servo" {
            w278 = FALSE ("Visible")
            n145 = call <vilib>:"NT Read Number.vi"("Name"=w280) -> ("Numeric"=w279:dbl)  [unwired: 9 in, 1 out]
            n146 = property on="Test Slider" class="Slide (strict)"("Visible"=TRUE, "Scale.Maximum"=170.0 ("Scale.Range:Maximum")) -> ()  [unwired: 2 in, 2 out]
            n147 = local write "Test Slider"(w279) -> ()
            n148 = property on="Motor" class="Clust (strict)"("Visible"=w278) -> ()  [unwired: 2 in, 2 out]
            n149 = property on="Rev/Fwd" class="Clust (strict)"("Visible"=w278) -> ()  [unwired: 2 in, 2 out]
            n150 = property on="On/Off" class="Bool (strict)"("Visible"=w278) -> ()  [unwired: 2 in, 2 out]
            n151 = property on="Test Ring" class="Ring (strict)"("Visible"=w278) -> ()  [unwired: 2 in, 2 out]
          }
          frame "Relay", "Solenoid" {
            w281 = FALSE ("Visible")
            n152 = property on="Motor" class="Clust (strict)"("Visible"=w281) -> ()  [unwired: 2 in, 2 out]
            n153 = property on="Test Slider" class="Slide (strict)"("Visible"=w281) -> ()  [unwired: 2 in, 2 out]
            n154 = Search and Replace String(input string=w282, search string="/Value  **", replace string="/Direction") -> (result string=w288:string)  [unwired: 5 in, 3 out]
            n155 = property on="Test Ring" class="Ring (strict)"("Visible"=w281) -> ()  [unwired: 2 in, 2 out]
            n156 = call <vilib>:"NT Read String.vi"("Name"=w288) -> ("String"=w286:string)  [unwired: 9 in, 1 out]
            n157 = Equal?(x="Both directions", y=w286) -> (x = y?=w284:bool)
            n158 = Not(x=w284) -> (.not. x?=w285:bool)
            n159 = property on="Rev/Fwd" class="Clust (strict)"("Visible"=w284) -> ()  [unwired: 2 in, 2 out]
            n160 = property on="On/Off" class="Bool (strict)"("Visible"=w285, "Caption.Text"=w283) -> ()  [unwired: 2 in, 2 out]
          }
          frame "Compressor", "Digital Out" {
            w291 = FALSE ("Visible")
            # "Get direction and finish"
            n161 = property on="Motor" class="Clust (strict)"("Visible"=w291) -> ()  [unwired: 2 in, 2 out]
            n162 = property on="Test Slider" class="Slide (strict)"("Visible"=w291) -> ()  [unwired: 2 in, 2 out]
            n163 = property on="Test Ring" class="Ring (strict)"("Visible"=w291) -> ()  [unwired: 2 in, 2 out]
            n164 = property on="On/Off" class="Bool (strict)"("Visible"=TRUE, "Caption.Text"=w292) -> ()  [unwired: 2 in, 2 out]
            n165 = property on="Rev/Fwd" class="Clust (strict)"("Visible"=FALSE) -> ()  [unwired: 2 in, 2 out]
          }
          frame "Camera" {
            n166 = call <vilib>:"Get Last Path Segment.vi"("String in"=w299) -> ("String out"=w300:string)  [unwired: 10 in]
            n167 = property on="On/Off" class="Bool (strict)"("Visible"=FALSE) -> ()  [unwired: 2 in, 2 out]
            n168 = property on="Motor" class="Clust (strict)"("Visible"=FALSE) -> ()  [unwired: 2 in, 2 out]
            n169 = property on="Rev/Fwd" class="Clust (strict)"("Visible"=FALSE) -> ()  [unwired: 2 in, 2 out]
            n170 = case shown="\"White Balance  **\"" w300 {
              tunnel: w299 -> [w306 w315 w324 w333 w342 _ w348]
              tunnel: w298 -> [w304 w312 w321 w330 w339 _ _]
              frame "Size  **" {
                n171 = Index Array(array=w304) -> (element=w303:cluster{string[]})  [unwired: 1 in]
                n172 = call <vilib>:"NT Read String.vi"("Name"=w306) -> ("String"=w305:string)  [unwired: 9 in, 1 out]
                n173 = Unbundle(w303) -> (w301:string[])
                n174 = Match First String(2:w301, 3:w305) -> (0:w302:i32)  [unwired: 1 out]
                n175 = property on="Test Ring" class="Ring (strict)"("Value"=w302, "Strings []"=w301) -> ()  [unwired: 2 in, 2 out]
                n176 = property on="Test Ring" class="Ring (strict)"("Visible"=TRUE) -> ()  [unwired: 2 in, 2 out]
                n177 = property on="Test Slider" class="Slide (strict)"("Visible"=FALSE) -> ()  [unwired: 2 in, 2 out]
              }
              frame "White Balance  **" {
                n178 = Index Array(array=w312, index=1) -> (element=w313:cluster{string[]})
                n179 = call <vilib>:"NT Read String.vi"("Name"=w315) -> ("String"=w314:string)  [unwired: 9 in, 1 out]
                n180 = Unbundle(w313) -> (w310:string[])
                n181 = Match First String(2:w310, 3:w314) -> (0:w309:i32)  [unwired: 1 out]
                n182 = property on="Test Ring" class="Ring (strict)"("Value"=w309, "Strings []"=w310) -> ()  [unwired: 2 in, 2 out]
                n183 = property on="Test Ring" class="Ring (strict)"("Visible"=TRUE) -> ()  [unwired: 2 in, 2 out]
                n184 = property on="Test Slider" class="Slide (strict)"("Visible"=FALSE) -> ()  [unwired: 2 in, 2 out]
              }
              frame "Exposure  **" {
                n185 = Index Array(array=w321, index=2) -> (element=w322:cluster{string[]})
                n186 = call <vilib>:"NT Read String.vi"("Name"=w324) -> ("String"=w323:string)  [unwired: 9 in, 1 out]
                n187 = Unbundle(w322) -> (w318:string[])
                n188 = Match First String(2:w318, 3:w323) -> (0:w319:i32)  [unwired: 1 out]
                n189 = property on="Test Ring" class="Ring (strict)"("Value"=w319, "Strings []"=w318) -> ()  [unwired: 2 in, 2 out]
                n190 = property on="Test Ring" class="Ring (strict)"("Visible"=TRUE) -> ()  [unwired: 2 in, 2 out]
                n191 = property on="Test Slider" class="Slide (strict)"("Visible"=FALSE) -> ()  [unwired: 2 in, 2 out]
              }
              frame "Exposure Priority  **" {
                n192 = Index Array(array=w330, index=3) -> (element=w331:cluster{string[]})
                n193 = call <vilib>:"NT Read String.vi"("Name"=w333) -> ("String"=w332:string)  [unwired: 9 in, 1 out]
                n194 = Unbundle(w331) -> (w327:string[])
                n195 = Match First String(2:w327, 3:w332) -> (0:w328:i32)  [unwired: 1 out]
                n196 = property on="Test Ring" class="Ring (strict)"("Value"=w328, "Strings []"=w327) -> ()  [unwired: 2 in, 2 out]
                n197 = property on="Test Ring" class="Ring (strict)"("Visible"=TRUE) -> ()  [unwired: 2 in, 2 out]
                n198 = property on="Test Slider" class="Slide (strict)"("Visible"=FALSE) -> ()  [unwired: 2 in, 2 out]
              }
              frame "Color Enable  **" {
                n199 = Index Array(array=w339, index=4) -> (element=w340:cluster{string[]})
                n200 = call <vilib>:"NT Read String.vi"("Name"=w342) -> ("String"=w341:string)  [unwired: 9 in, 1 out]
                n201 = Unbundle(w340) -> (w336:string[])
                n202 = Match First String(2:w336, 3:w341) -> (0:w337:i32)  [unwired: 1 out]
                n203 = property on="Test Ring" class="Ring (strict)"("Value"=w337, "Strings []"=w336) -> ()  [unwired: 2 in, 2 out]
                n204 = property on="Test Ring" class="Ring (strict)"("Visible"=TRUE) -> ()  [unwired: 2 in, 2 out]
                n205 = property on="Test Slider" class="Slide (strict)"("Visible"=FALSE) -> ()  [unwired: 2 in, 2 out]
              }
              frame Default {
                n206 = property on="Test Ring" class="Ring (strict)"("Visible"=FALSE) -> ()  [unwired: 2 in, 2 out]
                n207 = property on="Test Slider" class="Slide (strict)"("Visible"=FALSE) -> ()  [unwired: 2 in, 2 out]
              }
              frame "Brightness  **", "Color Level  **", "Compression  **", "FPS  **", "Sharpness  **" {
                n208 = call <vilib>:"NT Read Number.vi"("Name"=w348) -> ("Numeric"=w347:dbl)  [unwired: 9 in, 1 out]
                n209 = local write "Test Slider"(w347) -> ()
                n210 = property on="Test Slider" class="Slide (strict)"("Visible"=TRUE, "Scale.Maximum"=100.0 ("Scale.Range:Maximum")) -> ()  [unwired: 2 in, 2 out]
                n211 = property on="Test Ring" class="Ring (strict)"("Visible"=FALSE) -> ()  [unwired: 2 in, 2 out]
              }
            }
          }
        }
        n212 = property on="Progress" class="Clust (strict)"("Visible"=FALSE) -> ()  [unwired: 2 in, 2 out]
      }
      event "Test Name": Mouse Enter {
        # "Populate the ring with the list of tests"
        n213 = event-data() -> ()  [unwired: 1 in, 1 out]
        n214 = call <vilib>:"NT Read String Array.vi"("Name"="TestMode/TestList") -> ("String Array"=w356:string[])  [unwired: 9 in, 1 out]
        n215 = Build Array (concatenate)("Select the test to run...", w356) -> (w355:string[])
        n216 = property on="Test Name" class="Ring (strict)"("Strings []"=w355) -> ()  [unwired: 2 in, 2 out]
      }
      event "Test Name": Value Change {
        w358 = FALSE ("Visible")
        # "Tell the robot the test name to run"
        n217 = event-data() -> ("NewVal"=w362:u16)  [unwired: 1 in]
        n218 = property on="Test Name" class="Ring (strict)"() -> ("Strings []"=w363:string[])  [unwired: 2 in, 2 out]
        n219 = local write "Progress"(T10 {"Test Progress"=0, "Test Progress Text"=""} ("Progress")) -> ()
        n220 = Index Array(array=w363, index=w362) -> (element=w361:string)
        n221 = call <vilib>:"NT Write String.vi"("String"=w361, "Name"="TestMode/TestName") -> ()  [unwired: 9 in, 1 out]
        n222 = property on="Progress" class="Clust (strict)"("Visible"=TRUE) -> ()  [unwired: 2 in, 2 out]
        n223 = property on="Motor" class="Clust (strict)"("Visible"=w358) -> ()  [unwired: 2 in, 2 out]
        n224 = property on="Test Slider" class="Slide (strict)"("Visible"=w358) -> ()  [unwired: 2 in, 2 out]
        n225 = property on="On/Off" class="Bool (strict)"("Visible"=w358) -> ()  [unwired: 2 in, 2 out]
        n226 = property on="Rev/Fwd" class="Clust (strict)"("Visible"=w358) -> ()  [unwired: 2 in, 2 out]
        n227 = property on="Test Ring" class="Ring (strict)"("Visible"=w358) -> ()  [unwired: 2 in, 2 out]
      }
      event "Listbox": Double Click {
        n228 = event-data() -> ("PlatMods.Shift"=w366:bool, "Row"=w368:i32)  [unwired: 1 in]
        n229 = case shown="True" w366 {
          tunnel: w368 -> [w372 _]
          tunnel: 1 -> [w371 _]
          frame False {
            n230 = property on="Listbox" class="LstBox (strict)"() -> ("Item Symbols"=w370:i32[])  [unwired: 2 in, 2 out]
            n231 = Replace Array Subset(array=w370, new element=w371, index=w372) -> (w369:i32[])
            n232 = property on="Listbox" class="LstBox (strict)"("Item Symbols"=w369) -> ()  [unwired: 2 in, 2 out]
          }
          frame True {
            w373 = 0 ("Top Row")
            n233 = property on="Listbox" class="LstBox (strict)"() -> ("Number of Rows"=w375:u32)  [unwired: 2 in, 2 out]
            n234 = Initialize Array(0, w375) -> (w374:i32[])
            n235 = property on="Listbox" class="LstBox (strict)"("Top Row"=w373, "Value"=w373, "Item Symbols"=w374) -> ()  [unwired: 2 in, 2 out]
          }
        }
      }
      event "Listbox": Key Down {
        n236 = event-data() -> ("VKey"=w379:T23)  [unwired: 1 in]
        n237 = case shown="\"Left\", \"Right\"" w379 {
          selector: w379 -> [w384 _]
          tunnel: eventvkey."Left" ("VKey") -> [w382 _]
          frame "Left", "Right" {
            n238 = Equal?(x=w382, y=w384) -> (x = y?=w383:bool)
            n239 = Select(t=0, s=w383, f=1) -> (s? t:f=w385:i32)
            n240 = property on="Listbox" class="LstBox (strict)"() -> ("Item Symbols"=w388:i32[])  [unwired: 2 in, 2 out]
            n241 = Replace Array Subset(array=w388, new element=w385, index="Listbox") -> (w387:i32[])
            n242 = property on="Listbox" class="LstBox (strict)"("Item Symbols"=w387) -> ()  [unwired: 2 in, 2 out]
          }
          frame Default {
          }
        }
      }
      event "DB Camera Config": Value Change {
        n243 = event-data() -> ("NewVal"=w392:bool)  [unwired: 1 in]
        n244 = case shown="False" w392 {
          tunnel: w391 -> [w401 _]
          tunnel: [w394 w412] -> w390
          tunnel: w389 -> [w393 w412]
          frame False {
            w408 = "Camera"
            w411 = FALSE ("Visible")
            n245 = local read "Camera Settings"() -> (w400:T2)
            n246 = Index Array(array=w401) -> (element=w404:cluster{string[]})  [unwired: 1 in]
            n247 = Unbundle(w400) -> ("Frame Rate"=w399:i32, "Compression"=w398:i32, "Size"=w402:u16)
            n248 = Unbundle(w404) -> (w403:string[])
            n249 = Index Array(array=w403, index=w402) -> (element=w397:string)
            n250 = call-poly <vilib>:"Write Key.vi"("section"=w408, "value"=w397, "key"="Size", "refnum"=w393) -> ("refnum out"=w410:T22)  [unwired: 2 in, 5 out]
            n251 = call-poly <vilib>:"Write Key.vi"("section"=w408, "value"=w399, "key"="FrameRate", "refnum"=w410) -> ("refnum out"=w409:T22)  [unwired: 1 in, 6 out]
            n252 = property on="Camera Settings" class="Clust (strict)"("Visible"=w411) -> ()  [unwired: 2 in, 2 out]
            n253 = local write "DB Camera Config"(w411) -> ()
            n254 = call-poly <vilib>:"Write Key.vi"("section"=w408, "value"=w398, "key"="Compression", "refnum"=w409) -> ("refnum out"=w395:T22)  [unwired: 1 in, 6 out]
            n255 = call <vilib>:"Close Config Data.vi"("refnum"=w395) -> ("file path"=w396:path)  [unwired: 2 in, 8 out]
            n256 = call <vilib>:"Open Config Data.vi"("configuration file path"=w396) -> ("refnum"=w394:T22)  [unwired: 8 in, 2 out]
          }
          frame True {
            n257 = property on="Camera Settings" class="Clust (strict)"("Visible"=TRUE) -> ()  [unwired: 2 in, 2 out]
          }
        }
      }
      event "Camera Settings": Value Change {
        n258 = event-data() -> ("NewVal"=w425:T2)  [unwired: 1 in]
        n259 = Index Array(array=w421) -> (element=w420:cluster{string[]})  [unwired: 1 in]
        n260 = Unbundle(w425) -> ("Frame Rate"=w416:i32, "Compression"=w415:i32, "Size"=w418:u16)
        n261 = Unbundle(w420) -> (w419:string[])
        n262 = Index Array(array=w419, index=w418) -> (element=w417:string)
        n263 = Format Into String(format string="%s   %dfps   %d%%", w417, w416, w415) -> (resulting string=w422:string)  [unwired: 2 in, 1 out]
        n264 = Build Array(w422) -> (w423:string[])
        n265 = property on="DB Camera Config" class="Bool (strict)"("Strings [4]"=w423) -> ()  [unwired: 2 in, 2 out]
      }
      event "Motor.Enable": Value Change {
        n266 = event-data() -> ("NewVal"=w431:bool)  [unwired: 1 in]
        n267 = Unbundle("Motor") -> ("Value"=w430:dbl)  [unwired: 1 out]
        n268 = Select(t=w430, s=w431, f=0.0) -> (s? t:f=w428:dbl)
        n269 = call <vilib>:"NT Write Number.vi"("Numeric"=w428, "Name"=w427) -> ()  [unwired: 9 in, 1 out]
      }
      event "Test Slider": Value Change {
        n270 = event-data() -> ("NewVal"=w434:dbl)  [unwired: 1 in]
        n271 = call <vilib>:"NT Write Number.vi"("Numeric"=w434, "Name"=w435) -> ()  [unwired: 9 in, 1 out]
      }
      event "On/Off": Value Change {
        n272 = event-data() -> ("NewVal"=w439:bool)  [unwired: 1 in]
        n273 = Boolean To (0,1)(Boolean=w439) -> (0, 1=w438:i16)
        n274 = call <vilib>:"NT Write Number.vi"("Numeric"=w438, "Name"=w437) -> ()  [unwired: 9 in, 1 out]
      }
      event "Rev/Fwd": Value Change {
        n275 = event-data() -> ("NewVal.Forward"=w447:bool, "NewVal.Reverse"=w446:bool)  [unwired: 1 in]
        n276 = Boolean To (0,1)(Boolean=w447) -> (0, 1=w443:i16)
        n277 = Boolean To (0,1)(Boolean=w446) -> (0, 1=w445:i16)
        n278 = Negate(x=w445) -> (-x=w444:i16)
        n279 = Add(x=w443, y=w444) -> (x+y=w442:i16)
        n280 = call <vilib>:"NT Write Number.vi"("Numeric"=w442, "Name"=w441) -> ()  [unwired: 9 in, 1 out]
      }
      event "Test Ring": Value Change {
        n281 = event-data() -> ("NewVal"=w451:u16)  [unwired: 1 in]
        n282 = property on="Test Ring" class="Ring (strict)"() -> ("Strings []"=w452:string[])  [unwired: 2 in, 2 out]
        n283 = Index Array(array=w452, index=w451) -> (element=w450:string)
        n284 = call <vilib>:"NT Write String.vi"("String"=w450, "Name"=w449) -> ()  [unwired: 9 in, 1 out]
      }
      event "Rec Mode": Value Change {
        # "Update globals for recording mode and path to read log from.\nClear when logging and let NetworkTables set path for vision to\nuse."
        n285 = event-data() -> ("NewVal"=w462:enum32{"Stop", "Record", "Playback"})  [unwired: 1 in]
        n286 = global write "WPI_DashboardLogging Global.vi" "Logging Filename"(path "") -> ()
        n287 = case shown="\"Stop\", \"Record\"" w462 {
          tunnel: w461 -> [_ w464 w472]
          tunnel: [_ _ w471] -> w458
          tunnel: [_ _ w470] -> _
          tunnel: w456 -> [_ _ w468]
          tunnel: cluster{i32, i32} {-250, 170} -> [_ _ w467]
          tunnel: [_ _ T24 {"Image Size"=TRUE, "Image Type"=TRUE, "Pixel Value"=TRUE, "ROI Information"=TRUE, "Zoom Factor"=FALSE} ("Image Information Shown:All Elements")] -> w454
          tunnel: [_ _ TRUE ("Zoom Factor")] -> w453
          frame Default {
          }
          frame "Stop", "Record" {
            # "Place Window too"
            n288 = invoke class="VI" method="FP.Close"(reference=w464) -> (reference out=w463:refnum<vi>)  [unwired: 2 in, 2 out]
            n289 = invoke class="VI" method="Abort VI"(reference=w463) -> ()  [unwired: 2 in, 3 out]
          }
          frame "Playback" {
            n290 = call "Open Playback Panel.vi"("Offset"=w467, "DB VI Ref"=w468, "Playback in"=w472) -> ("Playback out"=w469:refnum<vi>)  [unwired: 8 in]
            n291 = register-events(w469) -> (reference out=w471:refnum<event-registration>, error out=w470:errorcluster)  [unwired: 2 in]
          }
        }
        n292 = global write "WPI_DashboardLogging Global.vi" "Recording"(w462) -> ()
        n293 = property on="Camera Image" class="ImageControl"("Image Information Shown"=w454, "Image Information Visible"=w453) -> ()  [unwired: 2 in, 2 out]
        n294 = call <vilib>:"WPI_DashboardNT Log FieldName Cache.vi"("Operation"=enum16{"Lookup/Add", "Index", "Clear"}."Clear") -> ()  [unwired: 8 in, 3 out]
      }
      event Panel Close {
        w473 = enum32{"Stop", "Record", "Playback"}."Stop" ("Rec Mode")
        n295 = event-data() -> ()  [unwired: 1 in, 4 out]
        n296 = local write "Rec Mode"(w473) -> ()
        n297 = global write "WPI_DashboardLogging Global.vi" "Recording"(w473) -> ()
      }
      event Panel Close {
        # "Abort playback window and ourself"
        n298 = event-data() -> ()  [unwired: 1 in, 4 out]
        n299 = invoke class="VI" method="FP.Close"(reference=w478) -> (reference out=w477:refnum<vi>)  [unwired: 2 in, 2 out]
        n300 = invoke class="VI" method="Abort VI"(reference=w477) -> (error out=w476:errorcluster)  [unwired: 2 in, 2 out]
        n301 = invoke class="VI" method="Abort VI"(error in=w476) -> ()  [unwired: 2 in, 3 out]
      }
    }
  }
  n302 = property on="On/Off" class="Bool (strict)"("Visible"=w25) -> ()  [unwired: 2 in, 2 out]
  n303 = property on="Motor" class="Clust (strict)"("Visible"=w25) -> ()  [unwired: 2 in, 2 out]
  n304 = property on="Progress" class="Clust (strict)"("Visible"=w25) -> ()  [unwired: 2 in, 2 out]
  n305 = property on="Test Ring" class="Ring (strict)"("Visible"=w25) -> ()  [unwired: 2 in, 2 out]
  n306 = property on="Rev/Fwd" class="Clust (strict)"("Visible"=w25) -> ()  [unwired: 2 in, 2 out]
  n307 = property on="Camera Settings" class="Clust (strict)"("Visible"=w25) -> ()  [unwired: 2 in, 2 out]
  n308 = local write "DB Camera Config"(w25) -> ()
  n309 = global write "WPI_DashboardLogging Global.vi" "Recording"(w8) -> ()
  n310 = local write "Rec Mode"(w8) -> ()
